vi "set_speed.vi"(8 "error in (no error)":errorcluster caption="错误输入（无错误）", 10 "speed":i32, 11 "StepMotor 输入":refnum<class "StepMotor.lvclass">) -> (0 "error out":errorcluster caption="错误输出", 3 "StepMotor 输出":refnum<class "StepMotor.lvclass">)   [LabVIEW 2016, in "MotionControl_UFO_3DOF.lvlib" / "StepMotor.lvclass"]
uses:
  <userlib>/MotionControl_UFO_3DOF/StepMotor/StepMotor.lvclass
  <userlib>/MotionControl_UFO_3DOF/StepMotor/StepMotor.lvclass/StepMotor.ctl
  <userlib>/UISimCanFunc_wrapper/UISimCanFunc_wrapper.lvlib
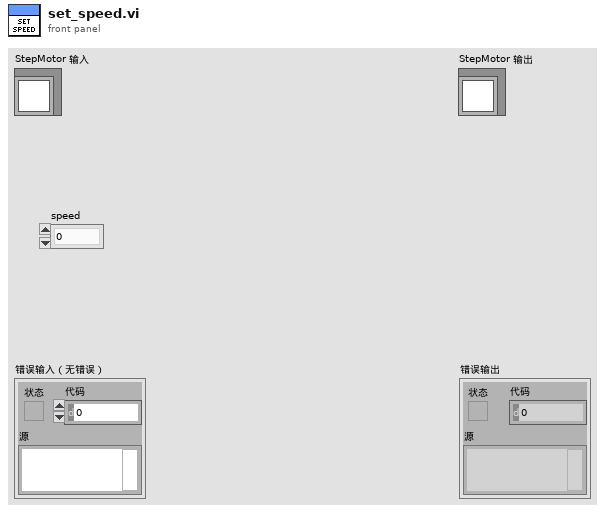
[diagram p1: front panel]
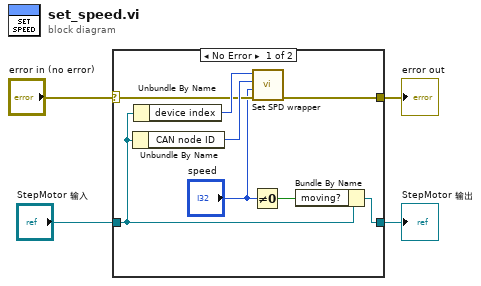
[diagram p0: block diagram]
diagram:
  n1 = case shown="No Error" "error in (no error)" {
    selector: "error in (no error)" -> [w10 w14]
    tunnel: [w9 w14] -> w3
    tunnel: [w7 w13] -> w1
    tunnel: "StepMotor 输入" -> [w8 w13]
    frame No Error {
      n2 = Unbundle By Name(w8) -> ("CAN node ID"=w11:u32)
      n3 = Unbundle By Name(w8) -> ("device index"=w12:u32)
      n4 = Not Equal To 0?(x="speed") -> (x != 0?=w5:bool)
      n5 = call <userlib>:"Set SPD wrapper.vi"("error in (no error)"=w10, "iValue"="speed", "dwCanNodeId"=w11, "dwDevIndex"=w12) -> ("error out"=w9:errorcluster)  [unwired: 5 in, 2 out]
      n6 = Bundle By Name(cluster=w8, "moving?"=w5) -> (w7:refnum<class "StepMotor.lvclass">)
    }
    frame Error {
    }
  }
  "error out" <- w3
  "StepMotor 输出" <- w1
